vi "Tegam4040 - Attenuation.vi"(0 "Instrument Session Handle In":u32 format="%x", 1 "Attenuation":T1(ring), 11 "error in (no error)":errorcluster) -> (4 "Instrument Session Handle Out (dupl)":u32 format="%x", 15 "error out":errorcluster)   [LabVIEW 2010, in "Tegam4040.lvlib"]
doc: "Attenuation Stage: Bits 2-4.\n\n0: Attenuator Stage not applied\n1: Attenuation of 1\n2: Attenuation of 10\n3: Attenuation of 100\n\nCalibration bit will be reset if attuation is changed."
uses:
  Tegam4040.lvlib
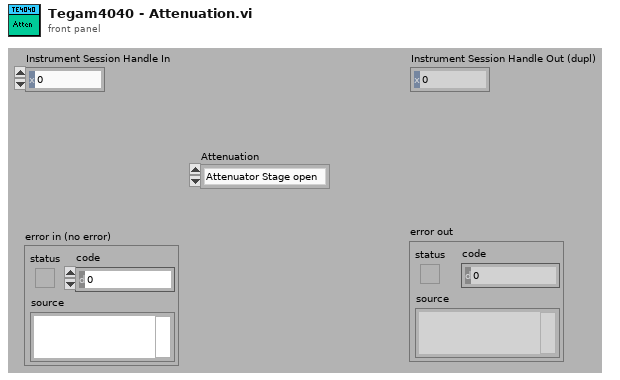
[diagram p1: front panel]
types:
  T1 = enum16{"Attenuator Stage open", "Attenuation of 1", "Attenuation of 10", "Attenuation of 100"}
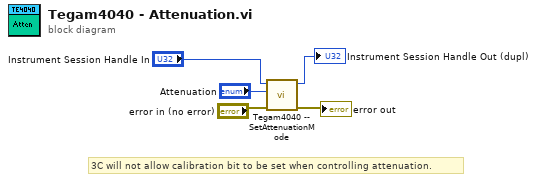
[diagram p0: block diagram]
diagram:
  # "3C will not allow calibration bit to be set when controlling attenuation."
  n1 = call "Tegam4040 -- SetAttenuationMode.vi"("error in (no error)"="error in (no error)", "Attenuation"="Attenuation", "Instrument Session Handle In"="Instrument Session Handle In") -> ("error out"=→"error out":errorcluster, "Instrument Session Handle Out (dupl)"=→"Instrument Session Handle Out (dupl)":u32)  [unwired: 7 in]
